vi "coloring2d.vi"(0 "?":u32[](array[colorbox])=[153, 16776960, 16711680], 1 "reference graph":refnum<vi>) -> ()   [LabVIEW 2015]
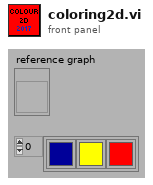
[diagram p1: front panel]
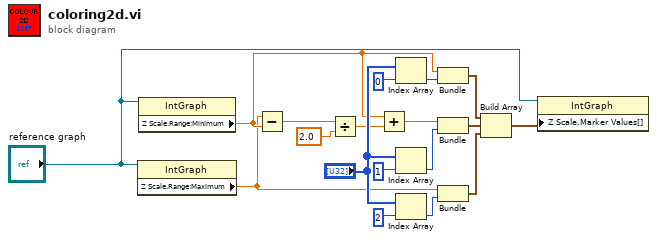
[diagram p0: block diagram]
diagram:
  n1 = property on="Property Node" class="IntGraph"(reference="reference graph") -> ("Z Scale.Range:Maximum"=w2:dbl)  [unwired: 1 in, 2 out]
  n2 = property on="Property Node" class="IntGraph"(reference="reference graph") -> ("Z Scale.Range:Minimum"=w4:dbl)  [unwired: 1 in, 2 out]
  n3 = Subtract(x=w2, y=w4) -> (x-y=w7:dbl)
  n4 = Divide(x=w7, y=2.0) -> (x/y=w5:dbl)
  n5 = Add(x=w4, y=w5) -> (x+y=w3:dbl)
  n6 = Index Array(array="?", index=0) -> (element=w14:u32)
  n7 = Index Array(array="?", index=1) -> (element=w13:u32)
  n8 = Index Array(array="?", index=2) -> (element=w12:u32)
  n9 = Bundle("ZScale.Minimum"=w4, w14) -> (w11:cluster{"ZScale.Minimum":dbl, u32})  [unwired: 1 out]
  n10 = Bundle(w3, w13) -> (w10:cluster{dbl, u32})  [unwired: 1 out]
  n11 = Bundle("ZScale.Maximum"=w2, w12) -> (w9:cluster{"ZScale.Maximum":dbl, u32})  [unwired: 1 out]
  n12 = Build Array(w11, w10, w9) -> (w8:cluster{"ZScale.Maximum":dbl, u32}[])
  n13 = property on="Property Node" class="IntGraph"(reference="reference graph", "Z Scale.Marker Values[]"=w8) -> ()  [unwired: 1 in, 2 out]
